vi "FlatToRichnidevice_grpc_IsReservedByClientResponse.vi"(5 "OutputClusterType":T1, 11 "InputCluster":T2) -> (3 "OutputCluster":T1)   [LabVIEW 2021, in "NI DAQmx_server.lvlib"]
uses:
  NI DAQmx_server.lvlib
  nidevice_grpc_IsReservedByClientResponse_Flat.ctl
  nidevice_grpc_IsReservedByClientResponse.ctl
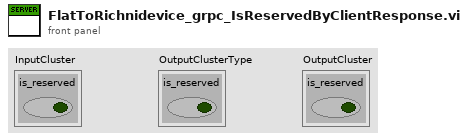
[diagram p1: front panel]
types:
  T1 = typedef "NI DAQmx_server.lvlib/nidevice_grpc_IsReservedByClientResponse.ctl" = cluster{"is_reserved":bool}
  T2 = typedef "NI DAQmx_server.lvlib/nidevice_grpc_IsReservedByClientResponse_Flat.ctl" = cluster{"is_reserved":bool}
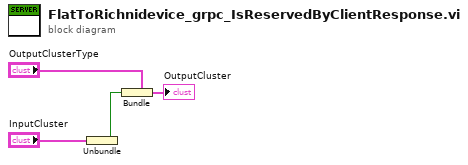
[diagram p0: block diagram]
diagram:
  n1 = Unbundle "Unbundle"("InputCluster") -> ("is_reserved"=w1:bool)
  n2 = Bundle "Bundle"(cluster="OutputClusterType", "is_reserved"=w1) -> (→"OutputCluster":T1)
